vi "Test Directory Prune and Create.vi"() -> (0 "error out":errorcluster, 3 "Pass":bool)   [LabVIEW 2021]
uses:
  <vilib>/Utility/error.llb/Clear Errors.vi
  <vilib>/Utility/libraryn.llb/Check if File or Folder Exists.vi
  File_CIF_U.lvlib
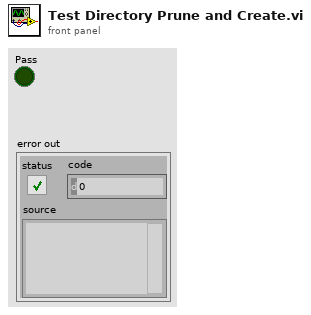
[diagram p1: front panel]
types:
  T1 = enum16{"open", "replace", "create", "open or create", "replace or create", "replace or create with confirmation"}
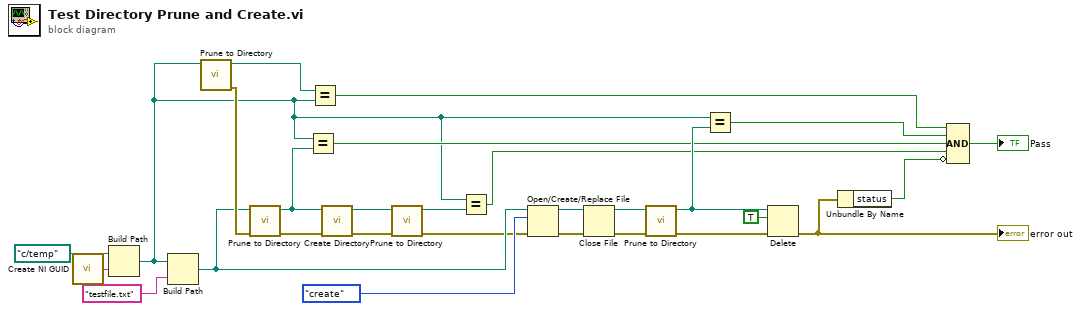
[diagram p0: block diagram]
diagram:
  n1 = call <vilib>:"Create NI GUID.vi"() -> ("NI GUID"=w25:string)
  n2 = Build Path(base path=path "c:/temp" ("Path In"), name or relative path=w25) -> (appended path=w2:path)
  n3 = Build Path(base path=w2, name or relative path="testfile.txt") -> (appended path=w21:path)
  n4 = call "Prune to Directory.vi"("Path In"=w2) -> ("error out"=w22:errorcluster, "Directory"=w23:path)  [unwired: 9 in]
  n5 = call "Prune to Directory.vi"("error in (no error)"=w22, "Path In"=w21) -> ("error out"=w28:errorcluster, "Directory"=w27:path)  [unwired: 8 in]
  n6 = Equal?(x=w2, y=w27) -> (x = y?=w10:bool)
  n7 = Equal?(x=w23, y=w2) -> (x = y?=w12:bool)
  n8 = call "Create Directory.vi"("error in (no error)"=w28, "Path In"=w27) -> ("error out"=w6:errorcluster, "Directory"=w4:path)  [unwired: 8 in]
  n9 = call "Prune to Directory.vi"("error in (no error)"=w6, "Path In"=w4) -> ("error out"=w5:errorcluster, "Directory"=w3:path)  [unwired: 8 in]
  n10 = Equal?(x=w2, y=w3) -> (x = y?=w1:bool)
  n11 = Open/Create/Replace File(file path (use dialog)=w21, error in=w5, operation (0:open)=T1."create") -> (refnum out=w17:refnum<file>, error out=w20:errorcluster)  [unwired: 3 in, 1 out]
  n12 = Close File(refnum=w17, error in=w20) -> (path=w18:path, error out=w19:errorcluster)
  n13 = call "Prune to Directory.vi"("error in (no error)"=w19, "Path In"=w18) -> ("error out"=w16:errorcluster, "Directory"=w15:path)  [unwired: 8 in]
  n14 = Equal?(x=w2, y=w15) -> (x = y?=w11:bool)
  n15 = Delete(path (use dialog)=w15, entire hierarchy (F)=TRUE, error in=w16) -> (error out=w13:errorcluster)  [unwired: 2 in, 2 out]
  "error out" <- w13
  n16 = Unbundle By Name(w13) -> ("status"=w7:bool)
  n17 = Compound Arithmetic op=AND(w12, w11, w10, w1, invert w7) -> (→"Pass":bool)
